vi "TriggerbasedProgramm1.vi"() -> ()   [LabVIEW 2022 SP3]
uses:
  <vilib>/DAQmx/create/channels.llb/DAQmx Create Channel (AI-Voltage-Basic).vi
  <vilib>/DAQmx/configure/timing.llb/DAQmx Timing (Sample Clock).vi
  <vilib>/DAQmx/configure/trigger.llb/DAQmx Start Trigger (Digital Edge).vi
  <vilib>/DAQmx/read.llb/DAQmx Read (Analog 1D Wfm NChan NSamp).vi
panel:
  in  "Stop Acquisition":bool
  in  "Trigger Mode":bool
  in  "File Name 2":string
  in  "Folder to save file to 2":path=path "A:/Source Localization/Material Evaluation paper/Dataset/Microphone Characterization/Clean Source"
  in  "physical channels 2":tag="cDAQ2Mod1/ai0, cDAQ2Mod1/ai3"
  in  "Sample Rate":dbl=200000.0 format="%0.2f"
  in  "Stop Visualization":bool
  out "?":dynamicdata(graph)=[{"t0"=timestamp(3806599236.6321588 s since 1904-01-01), "dt"=4.999999999999579e-07, "Y"=array[202167 elements], "attributes"=variant("NI_ChannelName"=variant(string "cDAQ2Mod1/ai0"), "NI_UnitDescription"=variant(string "Volts"))}]
  out "?":dynamicdata(graph)=[{"t0"=timestamp(3806599236.6321588 s since 1904-01-01), "dt"=4.999999999999579e-07, "Y"=array[202167 elements], "attributes"=variant("NI_ChannelName"=variant(string "cDAQ2Mod1/ai1"), "NI_UnitDescription"=variant(string "Volts"))}]
  in  "File Logging":bool
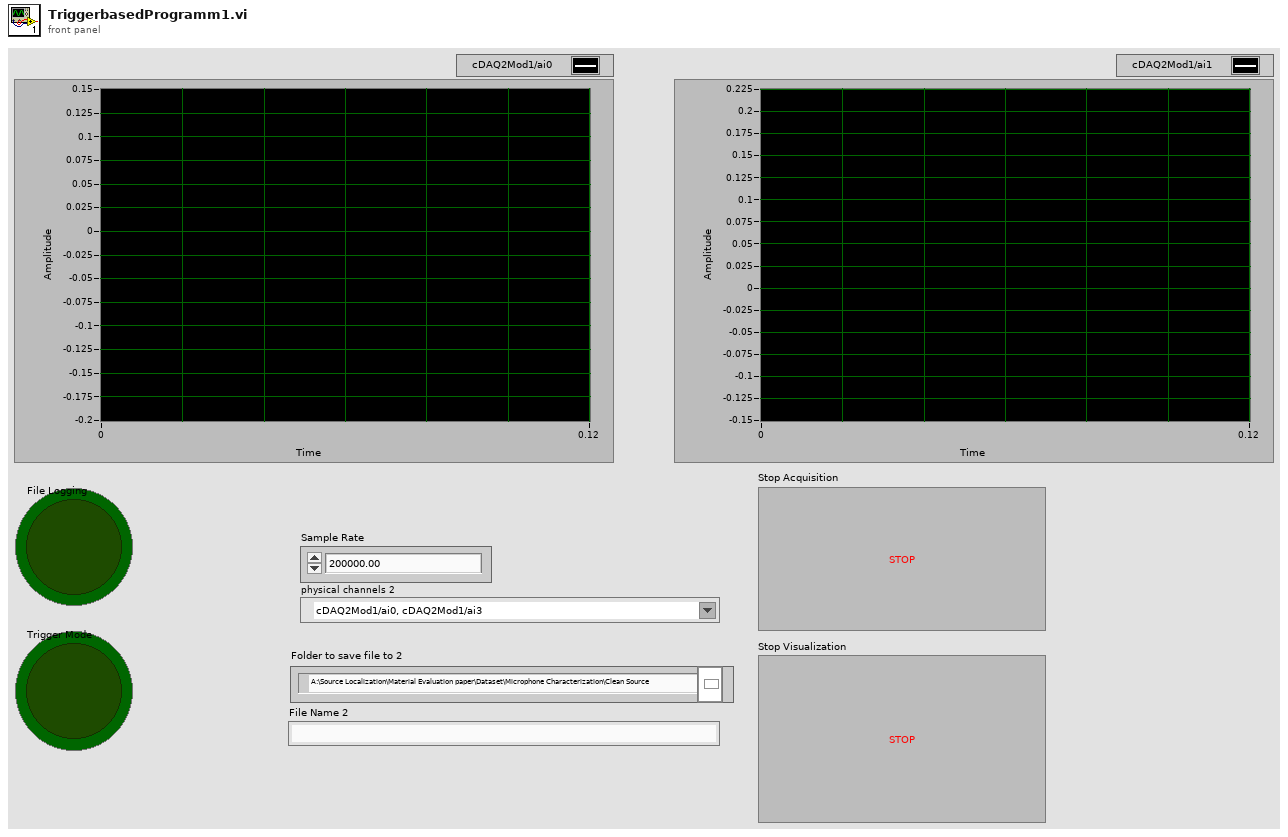
[diagram p1: front panel]
types:
  T1 = enum16{"open", "open or create", "create or replace", "create", "open (read-only)"}
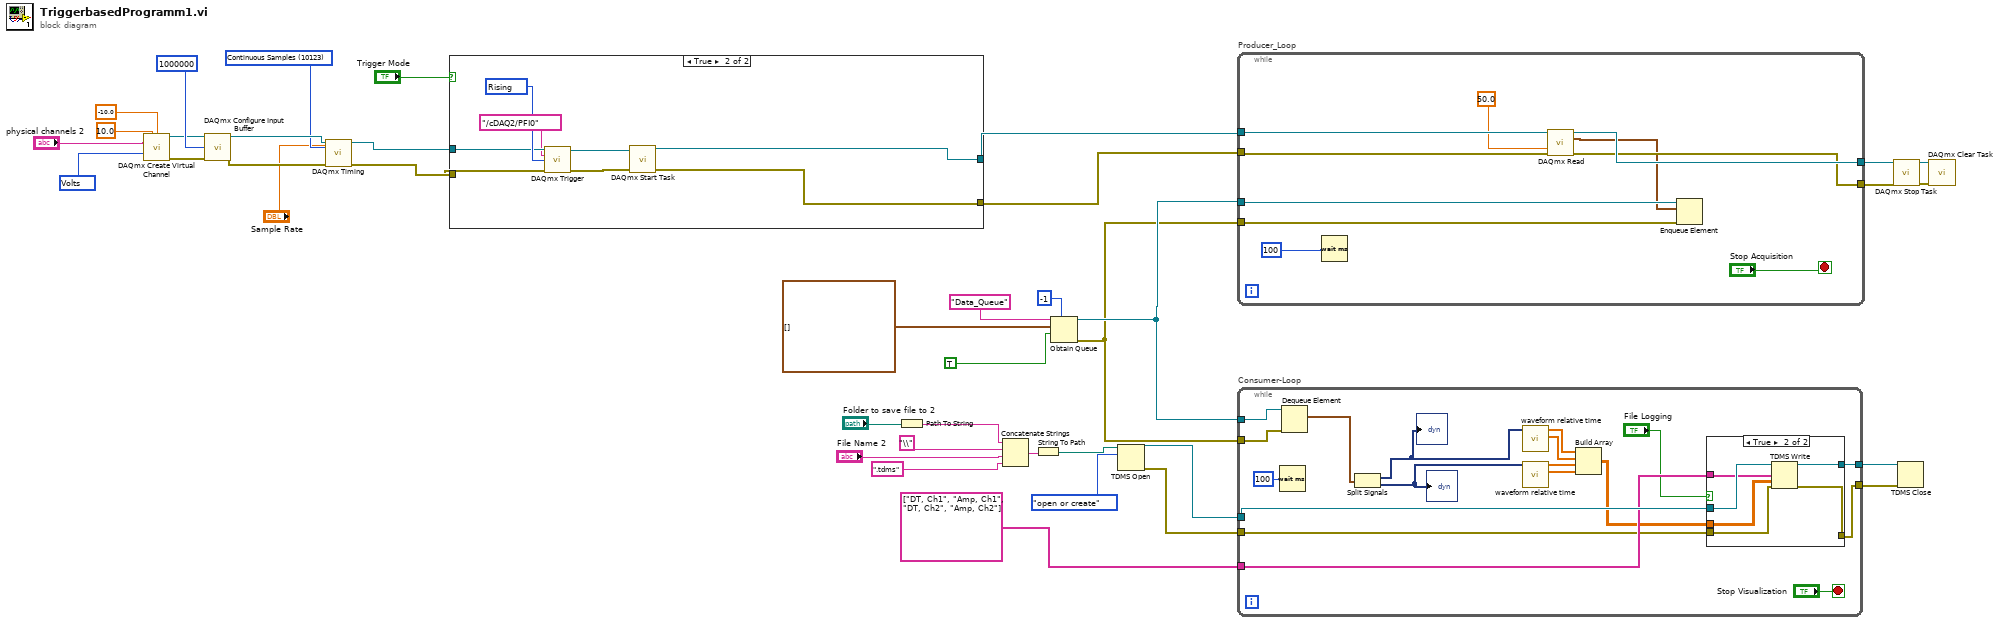
[diagram p0: block diagram]
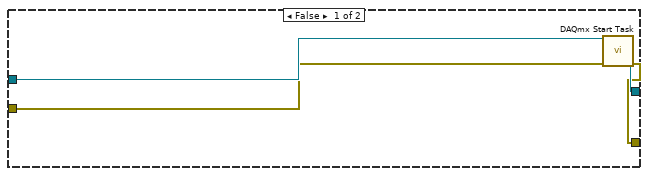
[diagram p2: hidden frame]
diagram:
  w11 = 10348 items=["Volts"=10348, "From Custom Scale"=10065] ("units")
  w35 = 10123 items=["Finite Samples"=10178, "Continuous Samples"=10123, "Hardware Timed Single Point"=12522] ("sample mode")
  n1 = call-poly <vilib>:"DAQmx Create Virtual Channel.vi"("maximum value"=10.0, "minimum value"=-10.0, "physical channels"="physical channels 2", "units"=w11) -> ("task out"=w2:refnum<k21>, "error out"=w39:errorcluster)  [unwired: 10 in]
  n2 = call <vilib>:"DAQmx Configure Input Buffer.vi"("task/channels in"=w2, "buffer size (in samples per channel)"=u32 1000000, "error in"=w39) -> ("task out"=w37:refnum<k21>, "error out"=w36:errorcluster)  [unwired: 11 in]
  n3 = call-poly <vilib>:"DAQmx Timing.vi"("task/channels in"=w37, "sample mode"=w35, "rate"="Sample Rate", "error in"=w36) -> ("task out"=w9:refnum<k21>, "error out"=w10:errorcluster)  [unwired: 10 in]
  n4 = case shown="True" "Trigger Mode" {
    tunnel: w10 -> [w41 w51]
    tunnel: w9 -> [w42 w47]
    tunnel: [w43 w45] -> w6
    tunnel: [w40 w46] -> w5
    frame False {
      n5 = call <vilib>:"DAQmx Start Task.vi"("task/channels in"=w42, "error in"=w41) -> ("task out"=w43:refnum<k21>, "error out"=w40:errorcluster)  [unwired: 12 in]
    }
    frame True {
      w48 = 10280 items=["Rising"=10280, "Falling"=10171] ("edge")
      n6 = call-poly <vilib>:"DAQmx Trigger.vi"("task/channels in"=w47, "source"=tag "/cDAQ2/PFI0", "edge"=w48, "error in"=w51) -> ("task out"=w50:refnum<k21>, "error out"=w49:errorcluster)  [unwired: 10 in]
      n7 = call <vilib>:"DAQmx Start Task.vi"("task/channels in"=w50, "error in"=w49) -> ("task out"=w45:refnum<k21>, "error out"=w46:errorcluster)  [unwired: 12 in]
    }
  }
  n8 = Path To String(path="Folder to save file to 2") -> (string=w31:string)
  n9 = Concatenate Strings(w31, "\\" ("string"), "File Name 2", ".tdms" ("string")) -> (w30:string)
  n10 = String To Path(string=w30) -> (path=w27:path)
  n11 = Obtain Queue(max queue size (-1, unlimited)=-1, name (unnamed)="Data_Queue", element data type=waveform(dbl)[] [] ("waveform"), create if not found? (T)=TRUE) -> (queue out=w21:refnum<queue>, error out=w16:errorcluster)  [unwired: 1 in, 1 out]
  n12 = TDMS Open(10:T1."open or create" ("operation (0:open)"), 11:w27) -> (0:w19:errorcluster, 3:w20:refnum<k34>)  [unwired: 5 in]
  n13 = while "Producer_Loop" {
    tunnel: w6 -> [w59]
    tunnel: w5 -> [w58]
    tunnel: w21 -> [w61]
    tunnel: w16 -> [w60]
    tunnel: [w57] -> w18
    tunnel: [w56] -> w17
    stop <- "Stop Acquisition" stop-if-true
    n14 = Wait (ms)(milliseconds to wait=u32 100) -> ()  [unwired: 1 out]
    n15 = call-poly <vilib>:"DAQmx Read.vi"("task/channels in"=w59, "timeout"=50.0, "error in"=w58) -> ("task out"=w57:refnum<k21>, "data"=w55:waveform(dbl)[], "error out"=w56:errorcluster)  [unwired: 10 in]
    n16 = Enqueue Element(queue=w61, element=w55, error in (no error)=w60) -> ()  [unwired: 1 in, 3 out]
  }
  n17 = while "Consumer-Loop" {
    tunnel: w21 -> [w79]
    tunnel: w20 -> [w77]
    tunnel: w19 -> [w66]
    tunnel: w16 -> [w78]
    tunnel: string[] ["DT, Ch1", "Amp, Ch1", "DT, Ch2", "Amp, Ch2"] ("channel name(s) in (Untitled)") -> [w76]
    tunnel: [w68] -> w14
    tunnel: [w65] -> w7
    stop <- "Stop Visualization" stop-if-true
    n18 = Wait (ms)(milliseconds to wait=u32 100) -> ()  [unwired: 1 out]
    n19 = Dequeue Element(queue=w79, error in (no error)=w78) -> (element=w75:waveform(dbl)[])  [unwired: 1 in, 3 out]
    n20 = Split Signals(w75) -> (w67:dynamicdata, w70:dynamicdata)  [unwired: 2 in]
    "?" <- w67
    "?" <- w70
    n21 = call "waveform relative time.vi"("signal in"=w67) -> ("Y"=w71:dbl[], "Relative Time"=w72:dbl[])  [unwired: 7 in, 2 out]
    n22 = call "waveform relative time.vi"("signal in"=w70) -> ("Y"=w74:dbl[], "Relative Time"=w73:dbl[])  [unwired: 7 in, 2 out]
    n23 = Build Array(w72, w71, w73, w74) -> (w69:dbl[][])
    n24 = case shown="True" "File Logging" {
      tunnel: w77 -> [w80 w87]
      tunnel: w76 -> [_ w86]
      tunnel: w69 -> [_ w85]
      tunnel: [w80 w84] -> w68
      tunnel: w66 -> [w81 w83]
      tunnel: [w81 w82] -> w65
      frame False {
      }
      frame True {
        n25 = TDMS Write(0:w87, 7:w86, 9:w85, 11:w83) -> (4:w84:refnum<k34>, 15:w82:errorcluster)  [unwired: 2 in, 2 out]
      }
    }
  }
  n26 = call <vilib>:"DAQmx Stop Task.vi"("task/channels in"=w18, "error in"=w17) -> ("task out"=w26:refnum<k21>, "error out"=w25:errorcluster)  [unwired: 12 in]
  n27 = TDMS Close(8:w7, 11:w14) -> ()  [unwired: 2 out]
  n28 = call <vilib>:"DAQmx Clear Task.vi"("task in"=w26, "error in"=w25) -> ()  [unwired: 13 in, 1 out]
